vi "Queue Is Nested.vi"(10 "Alias":string, 11 "Base Queue Actor in":refnum<class "Base Queue Actor.lvclass">) -> (2 "Queue Is Nested?":bool)   [LabVIEW 2021, in "jettl.lvlib" / "Base Queue Actor.lvclass"]
uses:
  Base Queue Actor.lvclass
  Base Queue Actor.lvclass/Base Queue Actor.ctl
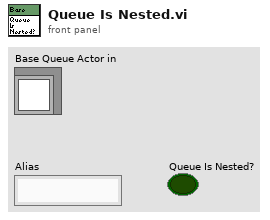
[diagram p1: front panel]
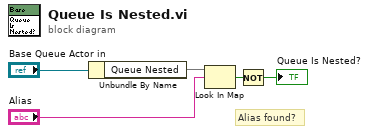
[diagram p0: block diagram]
diagram:
  # "Alias found?"
  n1 = Unbundle By Name("Base Queue Actor in") -> ("Queue Nested"=w4:map{string, refnum<data-value>})
  n2 = Look In Map(map=w4, key="Alias") -> (key not found?=w1:bool)  [unwired: 1 in, 1 out]
  n3 = Not(x=w1) -> (.not. x?=→"Queue Is Nested?":bool)
